vi "Revision Query Core.vi"(8 "error in (no error)":errorcluster, 11 "BNT_DAQmx-MCSV-RTD in":refnum<class "BNT_DAQmx-MCSV-RTD.lvclass">) -> (0 "error out":errorcluster, 1 "Firmware Revision":string, 2 "Driver Revision":string, 3 "BNT_DAQmx-MCSV-RTD out":refnum<class "BNT_DAQmx-MCSV-RTD.lvclass">)   [LabVIEW 2021, in "BNT_DAQmx.lvlib" / "BNT_DAQmx-MCSV-RTD.lvclass"]
uses:
  BNT_DAQmx-MCSV-RTD.lvclass
  BNT_DAQmx-MCSV/BNT_DAQmx-MCSV.lvclass
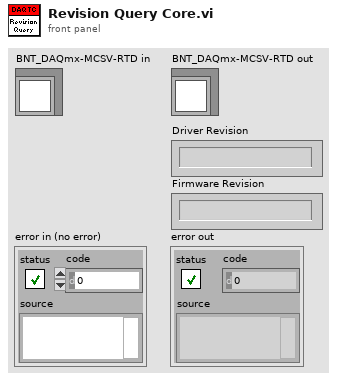
[diagram p1: front panel]
types:
  T1 = cluster{"Major":u16, "Minor":u16, "Fix":u16, "Build":u16}
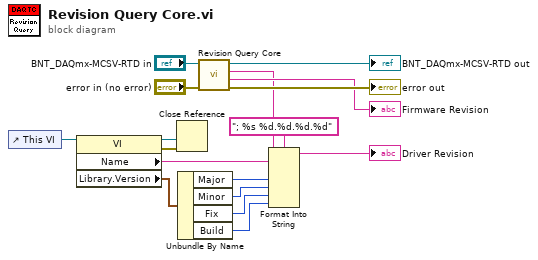
[diagram p0: block diagram]
diagram:
  n1 = control-ref of="This VI"() -> (w13:refnum<vi>)
  n2 = property class="VI"(reference=w13) -> (reference out=w11:refnum<vi>, error out=w12:errorcluster, "Name"=w4:string, "Library.Version"=w10:T1)  [unwired: 1 in]
  n3 = Close Reference(reference=w11, error in (no error)=w12) -> ()  [unwired: 1 out]
  n4 = Unbundle By Name(w10) -> ("Major"=w8:u16, "Minor"=w7:u16, "Fix"=w6:u16, "Build"=w5:u16)
  n5 = call-parent "Revision Query Core.vi"("error in (no error)"="error in (no error)", "BNT_DAQmx-MCSV in"="BNT_DAQmx-MCSV-RTD in") -> ("error out"=→"error out":errorcluster, "Firmware Revision"=→"Firmware Revision":string, "Driver Revision"=w2:string, "BNT_DAQmx-MCSV out"=→"BNT_DAQmx-MCSV-RTD out":refnum<class "BNT_DAQmx-MCSV-RTD.lvclass">)  [unwired: 6 in]
  n6 = Format Into String(format string="; %s %d.%d.%d.%d" ("Driver Revision"), initial string=w2, w4, w8, w7, w6, w5) -> (resulting string=→"Driver Revision":string)  [unwired: 1 in, 1 out]
